vi "get enumerate device information.vi"(8 "error in (no error)":errorcluster, 9 "device_information":T1, 10 "device_index":i32, 11 "device_enumeration":u64) -> (0 "error out":errorcluster, 1 "device_information out":T1, 3 "function return":i32)   [LabVIEW 2012, in "libximc.lvlib"]
doc: "result_t XIMC_API get_enumerate_device_information(device_enumeration_t device_enumeration, int device_index, device_information_t* device_information);"
uses:
  libximc.lvlib
  libximc.dll
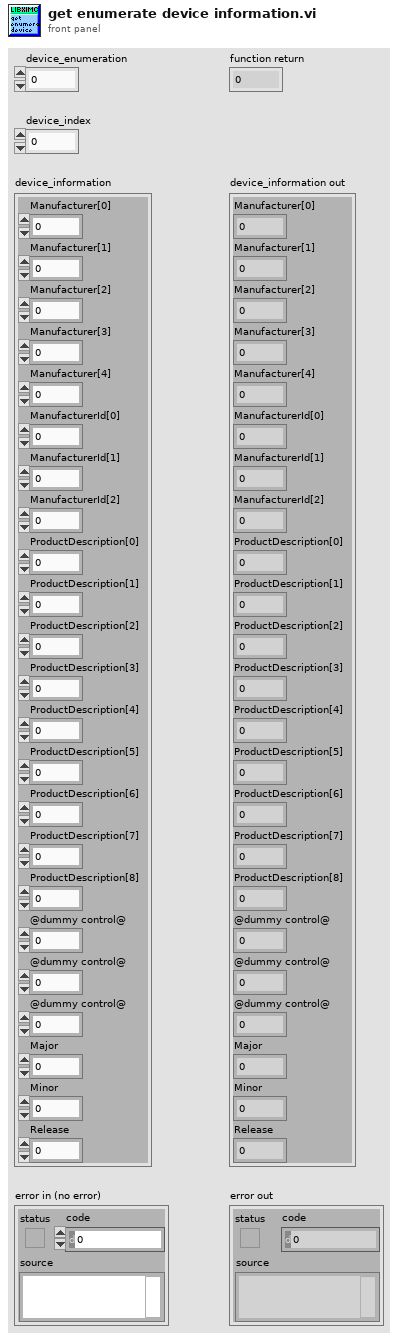
[diagram p1: front panel]
types:
  T1 = cluster{"Manufacturer[0]":i8, "Manufacturer[1]":i8, "Manufacturer[2]":i8, "Manufacturer[3]":i8, "Manufacturer[4]":i8, "ManufacturerId[0]":i8, "ManufacturerId[1]":i8, "ManufacturerId[2]":i8, "ProductDescription[0]":i8, "ProductDescription[1]":i8, "ProductDescription[2]":i8, "ProductDescription[3]":i8, "ProductDescription[4]":i8, "ProductDescription[5]":i8, "ProductDescription[6]":i8, "ProductDescription[7]":i8, "ProductDescription[8]":i8, "@dummy control@":i8, "@dummy control@":i8, "@dummy control@":i8, "Major":u32, "Minor":u32, "Release":u32}
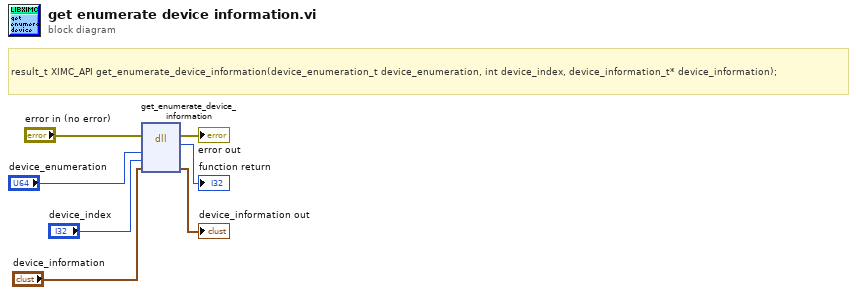
[diagram p0: block diagram]
diagram:
  # "result_t XIMC_API get_enumerate_device_information(device_enumeration_t device_enumeration, int device_index, device_information_t* device_information);"
  n1 = dll-call lib="C:/Users/Stepan/Downloads/labview_2.9.11_testgen_thread/libximc.*" fn="get_enumerate_device_information"(error in="error in (no error)", "device_enumeration"="device_enumeration", "device_index"="device_index", "device_information"="device_information") -> (error out=→"error out":errorcluster, →"function return":i32, "device_information"=→"device_information out":T1)  [unwired: 4 in, 1 out]
